vi "Tree Create.vi"(8 "error in (no error)":errorcluster, 10 "Shot":i32, 11 "Name":string) -> (0 "error out":errorcluster, 3 "Tree DVR out":refnum<data-value>)   [LabVIEW 2013, in "MDSplus.lvlib"]
uses:
  <vilib>/MDSplus/Library/MDSplus.lvlib
  <vilib>/MDSplus/Classes/Tree_Class/Tree.lvclass
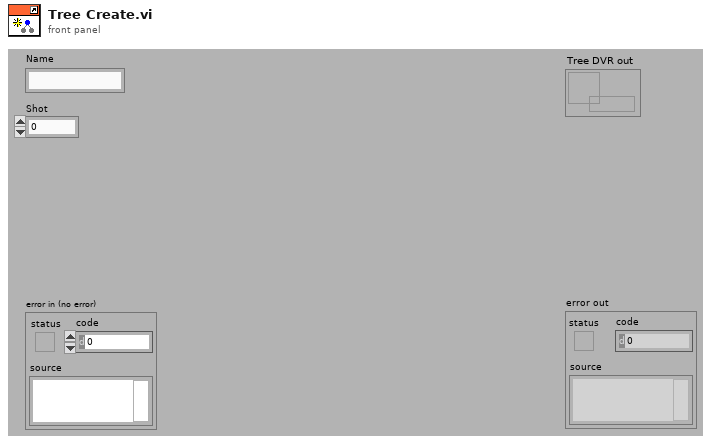
[diagram p1: front panel]
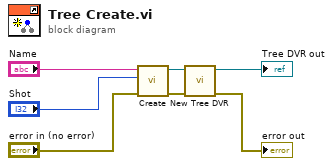
[diagram p0: block diagram]
diagram:
  n1 = call <vilib>:"Create.vi"("error in (no error)"="error in (no error)", "Shot"="Shot", "Name"="Name") -> ("error out"=w6:errorcluster, "Tree out"=w7:refnum<class "Tree.lvclass">)  [unwired: 7 in]
  n2 = call <vilib>:"New Tree DVR.vi"("error in (no error)"=w6, "Tree in"=w7) -> ("error out"=→"error out":errorcluster, "Tree DVR out"=→"Tree DVR out":refnum<data-value>)  [unwired: 8 in]
